vi "FarFieldCamera_param.vi"() -> ()   [LabVIEW 2018]
panel:
  in  "远场测量":bool
  in  "曝光时间/us":u32=10 min=10 step=1
  # "远场相机\n参数"
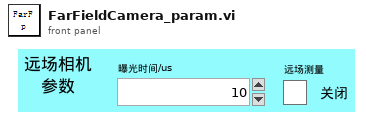
[diagram p1: front panel]
types:
  T1 = typedef "IMAQ Image.ctl" = refnum<image>
  T2 = cluster{"示波器":cluster{"Channel (0:Channel 1)":enum16{"Channel 1", "Channel 2", "Channel 3", "Channel 4"}, "电压范围":dbl, "触发电压":dbl, "时间范围":dbl, " 示波器VISA":refnum<visa-resource-name>, "时间范围 标签":u64, "电压范围 标签":u64, "触发电压 标签":u64, "输入阻抗/Ω":u64}, "光谱仪":cluster{"SpecDataReference":refnum<queue>, "grating center":dbl, "Exposure Time (s)":dbl, "是否进行详细设置":bool, " 开始通信检查":bool, "通信成功？":bool, "波长":dbl}, " 近场相机":cluster{"曝光时间/us":dbl, "模拟增益":i32, "控制套接字":i32, "IP 地址":string, " 采集套接字":i32, "  版本号":i32, "ImageData":T1, "  增益最大":i32, "  增益最小":i32, " 曝光最大":i32, " 曝光最小":i32, " 帧速":i32, " 同步切换":i32, "  曝光缩放":i32, "Camera Source":refnum<k21>, "近场X范围":dbl, "近场Y范围":dbl, "单个像元大小/um":dbl, "相机距离原点位置":dbl[], "是否测量发散角":bool, "光束类型":bool}, " 偏振仪":cluster{"电压范围":u64, "触发电压":u64, "时间范围":u64, "波长范围":enum16{"可见光 400-700nm", "近红外 700-1100nm"}, "可见光偏振测量仪VISA":refnum<visa-resource-name>, "近红外偏振测量仪VISA":refnum<visa-resource-name>}, " 功率计":cluster{"通道":enum16{"Channel 1", "Channel 2"}, "工作波长":u32, "单位":u64, "时间范围":u64, "IP地址":string, "端口":u32, "是否需要散射片":bool}, "能量计":cluster{"通道":enum16{"Channel 1", "Channel 2"}, "工作波长":u32, "单位":u64, "时间范围":u64, "IP地址":string, "端口":u32, "能量计量程":enum16{"200uJ", "20uJ", "2uJ", "200nJ"}}, "电机":cluster{"Channel (0:Channel 1)":enum16{"Channel 1", "Channel 2", "Channel 3", "Channel 4"}, "电压范围":u64, "触发电压":u64, "时间范围":u64}, " 远场相机":cluster{"曝光时间":i32, "模拟增益":i32, "控制套接字":i32, "IP 地址":string, " 采集套接字":i32, "  版本号":i32, "ImageData":T1, "  增益最大":i32, "  增益最小":i32, " 曝光最大":i32, " 曝光最小":i32, " 帧速":i32, " 同步切换":i32, "  曝光缩放":i32, "ImageData B":T1, "远场测量":bool}}
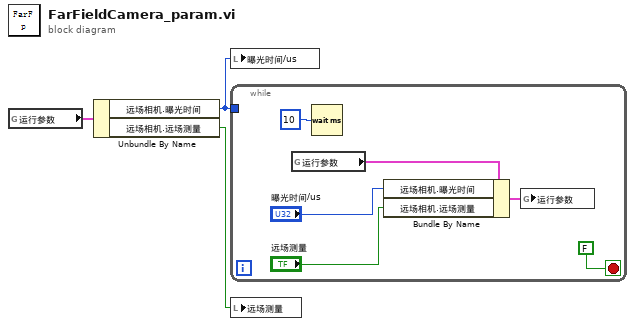
[diagram p0: block diagram]
diagram:
  n1 = global read "参数.vi" "运行参数"() -> (w3:T2)
  n2 = Unbundle By Name(w3) -> ("远场相机.曝光时间"=w2:i32, "远场相机.远场测量"=w1:bool)
  n3 = local write "曝光时间/us"(w2) -> ()
  n4 = while {
    tunnel: w2 -> [_]
    stop <- FALSE stop-if-true
    n5 = global read "参数.vi" "运行参数"() -> (w7:T2)
    n6 = Wait (ms)(milliseconds to wait=u32 10 ("等待时间（毫秒）")) -> ()  [unwired: 1 out]
    n7 = Bundle By Name(cluster=w7, "远场相机.曝光时间"="曝光时间/us", "远场相机.远场测量"="远场测量") -> (w6:T2)
    n8 = global write "参数.vi" "运行参数"(w6) -> ()
  }
  n9 = local write "远场测量"(w1) -> ()
